vi "Get Error Pointer.vi"(11 "Thread in":refnum<class "Thread.lvclass">) -> (2 "error pointer":refnum<class "Error Pointer.lvclass">, 3 "Thread out":refnum<class "Thread.lvclass">)   [LabVIEW 2020, in "DSF Core.lvlib" / "Thread.lvclass"]
uses:
  Thread.lvclass
  Pointers/Error/Error Pointer.lvclass
  Thread.lvclass/Thread.ctl
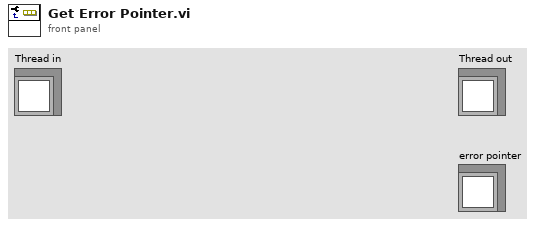
[diagram p1: front panel]
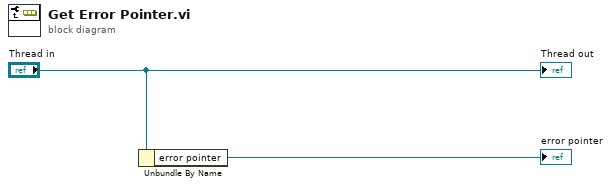
[diagram p0: block diagram]
diagram:
  n1 = Unbundle By Name("Thread in") -> ("error pointer"=→"error pointer":refnum<class "Error Pointer.lvclass">)
  "Thread out" <- "Thread in"
